vi "Apply Control Changes.vi"(7 "Type":enum16{"Control", "Indicator"}(ring), 9 "New":string[][](array[string]), 10 "Old":string[][](array[string]), 11 "Data In":T1[](array[typedef])) -> (1 "Changed Indices":i32[](array[numeric]), 3 "Data Out":T1[](array[typedef]))   [LabVIEW 2023, in "VI Properties Editor.lvlib"]
uses:
  CTLs/VI Data.ctl
  CTLs/VI Properties.ctl
  <vilib>/picture/picture.llb/imagedata.ctl
  CTLs/Control Properties.ctl
  VI Properties Editor.lvlib
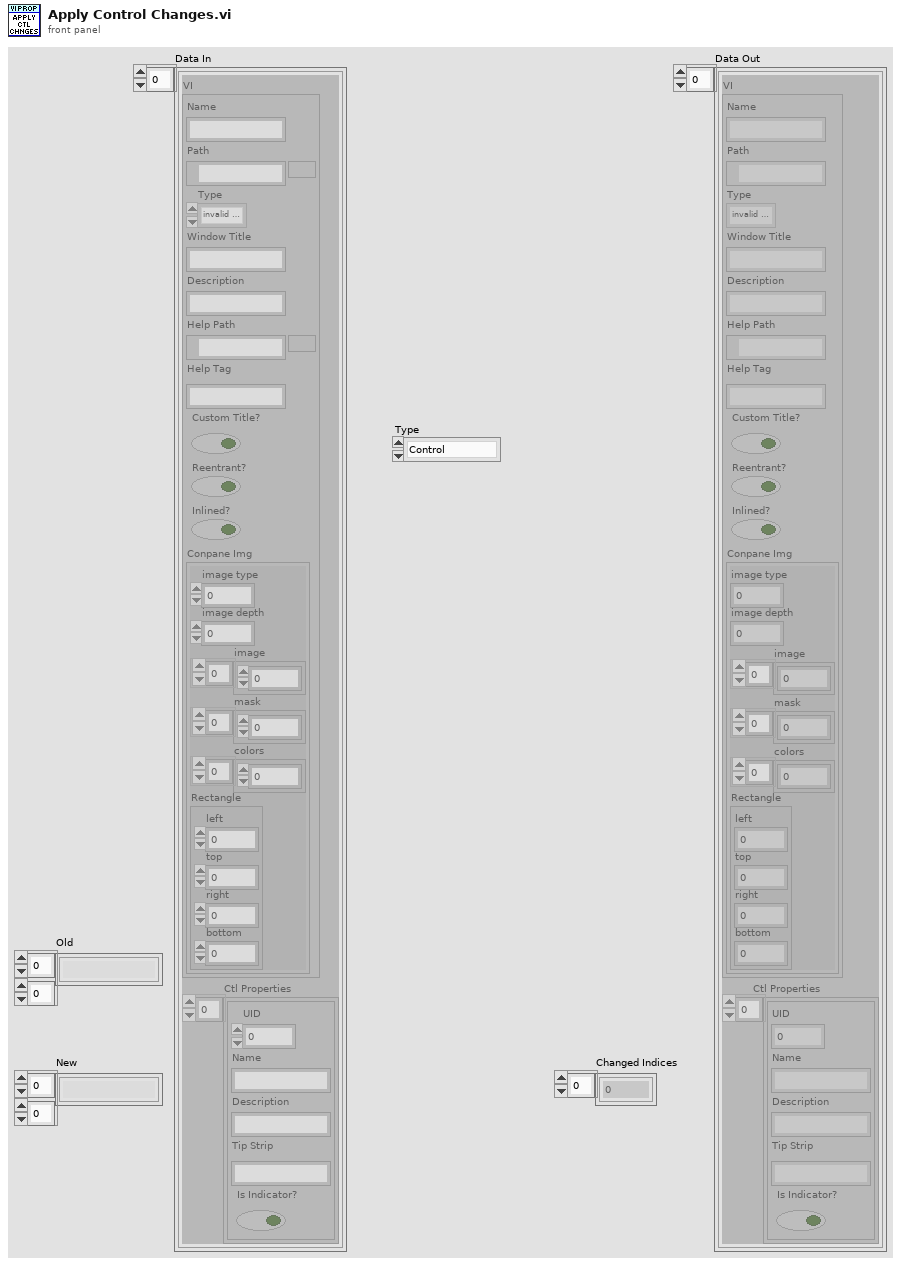
[diagram p1: front panel]
types:
  T1 = typedef "VI Properties Editor.lvlib/VI Data.ctl" = cluster{"VI":T2, "Ctl Properties":T4[]}
  T2 = typedef "VI Properties Editor.lvlib/VI Properties.ctl" = cluster{"Name":string, "Path":path, "Type":enum32{"invalid VI type", "Standard VI", "Control VI", "Global VI", "Polymorphic VI", "Configuration VI", "SubSystem", "Facade VI", "Method VI", "Statechart Diagram VI"}, "Window Title":string, "Description":string, "Help Path":path, "Help Tag":string, "Custom Title?":bool, "Reentrant?":bool, "Inlined?":bool, "Conpane Img":T3}
  T3 = typedef "imagedata.ctl" = cluster{"image type":i32, "image depth":i32, "image":u8[], "mask":u8[], "colors":u32[], "Rectangle":cluster{"left":i16, "top":i16, "right":i16, "bottom":i16}}
  T4 = typedef "VI Properties Editor.lvlib/Control Properties.ctl" = cluster{"UID":i32, "Name":string, "Description":string, "Tip Strip":string, "Is Indicator?":bool}
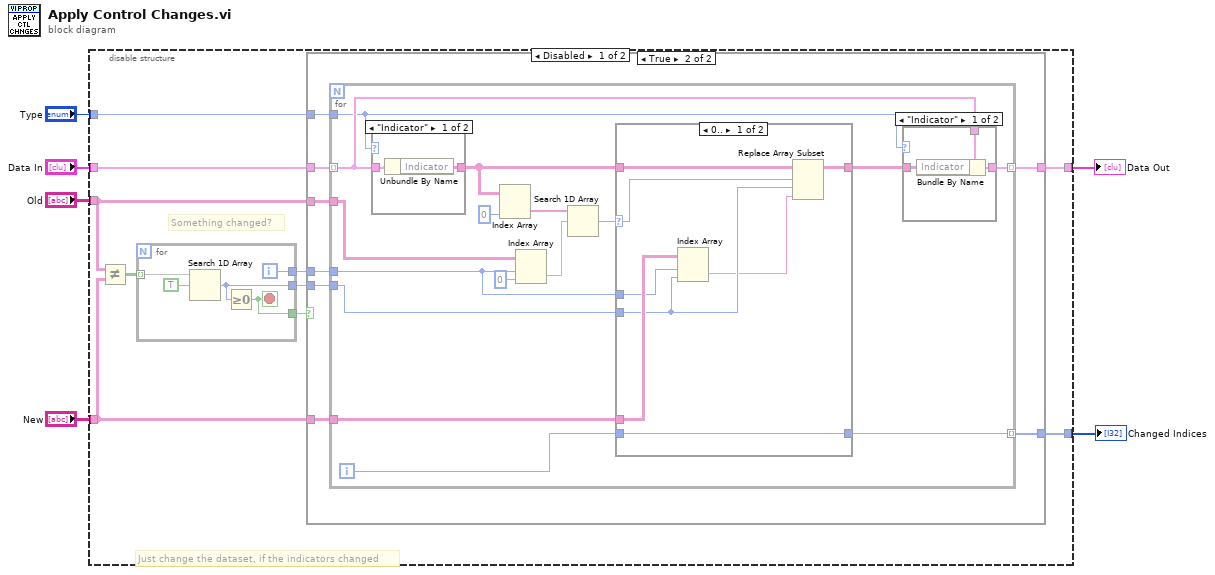
[diagram p0: block diagram]
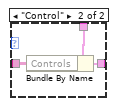
[diagram p3: hidden frame]
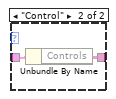
[diagram p4: hidden frame]
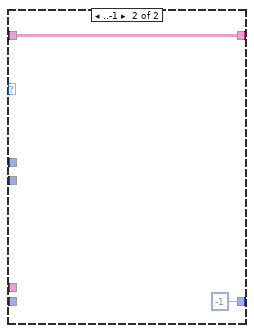
[diagram p5: hidden frame]
diagram:
  n1 = disable-structure shown="Disabled" {
    disable-tunnel: "Data In" -> [w15 _]
    disable-tunnel: [w14 _] -> w5
    disable-tunnel: "Old" -> [w13 _]
    disable-tunnel: "New" -> [w10 _]
    disable-tunnel: [w9 _] -> w2
    disable-tunnel: "Type" -> [w7 _]
    frame Disabled {
      # "Just change the dataset, if the indicators changed"
      # "Something changed?"
      n2 = Not Equal?(x=w13, y=w10) -> (x != y?=w16:bool[][])
      n3 = for {
        tunnel: w16 -> [w21] mode=indexing
        tunnel: [w19] -> w11
        tunnel: [w18] -> w12
        tunnel: [w17] -> w8
        i -> [w18]
        stop <- w17 stop-if-true
        n4 = Search 1D Array(1D array=w21, element=TRUE) -> (index of element=w19:i32)  [unwired: 1 in]
        n5 = Greater Or Equal To 0?(x=w19) -> (x >= 0?=w17:bool)
      }
      n6 = case shown="True" w8 {
        tunnel: w15 -> [w22 w30]
        tunnel: [w22 w26] -> w14
        tunnel: w13 -> [_ w29]
        tunnel: w12 -> [_ w28]
        tunnel: w11 -> [_ w27]
        tunnel: w10 -> [_ w25]
        tunnel: [_ w24] -> w9
        tunnel: w7 -> [_ w23]
        frame False {
        }
        frame True {
          n7 = for {
            tunnel: w30 -> [w34] mode=indexing
            tunnel: w29 -> [w44]
            tunnel: w28 -> [w38]
            tunnel: w27 -> [w40]
            tunnel: [w32] -> w26 mode=indexing
            tunnel: w25 -> [w39]
            tunnel: [w37] -> w24 mode=indexing
            tunnel: w23 -> [w31]
            i -> [w36]
            n8 = case shown="\"Indicator\"" w31 {
              tunnel: [w54 w56] -> w35
              tunnel: w34 -> [w53 w55]
              frame "Indicator" {
                n9 = Unbundle By Name(w53) -> ("Indicator"=w54:string[][])
              }
              frame "Control" {
                n10 = Unbundle By Name(w55) -> ("Controls"=w56:string[][])
              }
            }
            n11 = Index Array(array=w35, index (col)=0 ("disabled index (col)")) -> (element=w43:string[])  [unwired: 1 in]
            n12 = Index Array(array=w44, index (row)=w38, index (col)=0 ("disabled index (col)")) -> (element=w42:string)
            n13 = Search 1D Array(1D array=w43, element=w42) -> (index of element=w41:i32)  [unwired: 1 in]
            n14 = case shown="0.." w41 {
              selector: w41 -> [w58 _]
              tunnel: w35 -> [w64 w66]
              tunnel: [w63 w66] -> w33
              tunnel: w40 -> [w60 _]
              tunnel: w39 -> [w62 _]
              tunnel: w38 -> [w61 _]
              tunnel: [w57 -1 ("index of element")] -> w37
              tunnel: w36 -> [w57 _]
              frame 0.. {
                n15 = Index Array(array=w62, index (row)=w61, index (col)=w60) -> (element=w59:string)
                n16 = Replace Array Subset(array=w64, new element=w59, index (row)=w58, index (col)=w60) -> (w63:string[][])
              }
              frame ..-1 {
              }
            }
            n17 = case shown="\"Indicator\"" w31 {
              tunnel: w34 -> [w49 w52]
              tunnel: w33 -> [w48 w51]
              tunnel: [w47 w50] -> w32
              frame "Indicator" {
                n18 = Bundle By Name(cluster=w49, "Indicator"=w48) -> (w47:T1)
              }
              frame "Control" {
                n19 = Bundle By Name(cluster=w52, "Controls"=w51) -> (w50:T1)
              }
            }
          }
        }
      }
    }
    frame Enabled {
    }
  }
  "Data Out" <- w5
  "Changed Indices" <- w2
